vi "pp2_DAQwritePlayClick.vi"(0 "State In":T1={"Curr  tr"=0, "Curr (ms)"=0, "Cum (ms)"=0, "Run loop diff"=0, "Tone countdown (ms)"=0, "Countdown (ms)"=0, "Curr State"=enum."0 NULL", "Prev State"=enum."1 Habituation", "Null"=FALSE, "Sw"=FALSE, "Tone\nGate"=FALSE, "Stim"=FALSE, "Current DAQ DO Int"=0, "Current Loaded Trial"={"Trial Type Number"=1, "Trial Type"=enum."GO", "Trial Weight"=100, "Shock (mA)"=0.3, "Duration (ms)"=0.25, "Sound Type"=enum."04 FM Sweep", "Stim P1"=4000.0, "Stim P2"=0.0, "Stim P3"=0.0, "Stim P4"=2000.0}, "Next Trial (for display purposes)"={"Trial Type Number"=1, "Trial Type"=enum."GO", "Trial Weight"=100, "Shock (mA)"=0.3, "Duration (ms)"=0.25, "Sound Type"=enum."04 FM Sweep", "Stim P1"=4000.0, "Stim P2"=0.0, "Stim P3"=0.0, "Stim P4"=2000.0}, "Total trials memo"=0, "State start cum memo (ms)"=0, "Last dur jump time memo (ms)"=0, "Last dur shock time memo (ms)"=0, "Tone repeat memo (ms)"=0, "Webcam on"=FALSE, "Webcam recording"=FALSE} {"Current DAQ DO Int" format="%b"; "Next Trial (for display purposes)"."Shock (mA)" min=-1.0 max=5.0; "Next Trial (for display purposes)"."Trial Weight" step=1; "Next Trial (for display purposes)"."Duration (ms)" min=0.0 max=1.0; "Next Trial (for display purposes)"."Trial Type Number" min=1 step=1; "Current Loaded Trial"."Shock (mA)" min=-1.0 max=5.0; "Current Loaded Trial"."Trial Weight" step=1; "Current Loaded Trial"."Duration (ms)" min=0.0 max=1.0; "Current Loaded Trial"."Trial Type Number" min=1 step=1}, 1 "Daq config":T6={"Sound AO"="Dev2/ao0", "Shock intesity AO"="Dev1/ao1", "Code_LED DO"="Dev1/port1:2", "Switch DI"="Dev1/port0/line0:1", "Webcam"="cam0", "Sound AO task"="", "Sound card task"=0, "Shock intensity AO task"="", "Code_LED DO task"="", "Switch DI task"="", "AO <=> Sound card"=FALSE, "Sound card"=0, "sample rate"=8000.0, "Variable shock"=FALSE, "Webcam on"=FALSE, "Tone gate PFI"="/Dev1/PFI1", "Waveform memo"={"t0"=timestamp(0 s since 1904-01-01), "dt"=1.0, "Y"=[]}} {"sample rate" min=8000.0; "Sound card task" format="%.0x"}, 2 "Pre click \n(V)":dbl, 3 "error in (no error)":errorcluster) -> (8 "Daq config 2":T6={"Sound AO"="Dev2/ao0", "Shock intesity AO"="Dev1/ao1", "Code_LED DO"="Dev1/port1:2", "Switch DI"="Dev1/port0/line0:1", "Webcam"="cam0", "Sound AO task"="", "Sound card task"=0, "Shock intensity AO task"="", "Code_LED DO task"="", "Switch DI task"="", "AO <=> Sound card"=FALSE, "Sound card"=0, "sample rate"=8000.0, "Variable shock"=FALSE, "Webcam on"=FALSE, "Tone gate PFI"="/Dev1/PFI1", "Waveform memo"={"t0"=timestamp(0 s since 1904-01-01), "dt"=1.0, "Y"=[]}} {"sample rate" min=8000.0; "Sound card task" format="%.0x"}, 10 "error out":errorcluster)   [LabVIEW 2013]
uses:
  pp2_CTL_DaqConfig.ctl
  <vilib>/userdefined/High Color/IMAQdx.ctl
  <vilib>/sound2/lvsound2.llb/Sound Output Task ID.ctl
  pp2_CTL_StateInfo.ctl
  pp2_CTL_State.ctl
  pp2_Trial.ctl
  pp2_CTL_TrialType.ctl
  labolabo2/waveforms/WFTypes.ctl
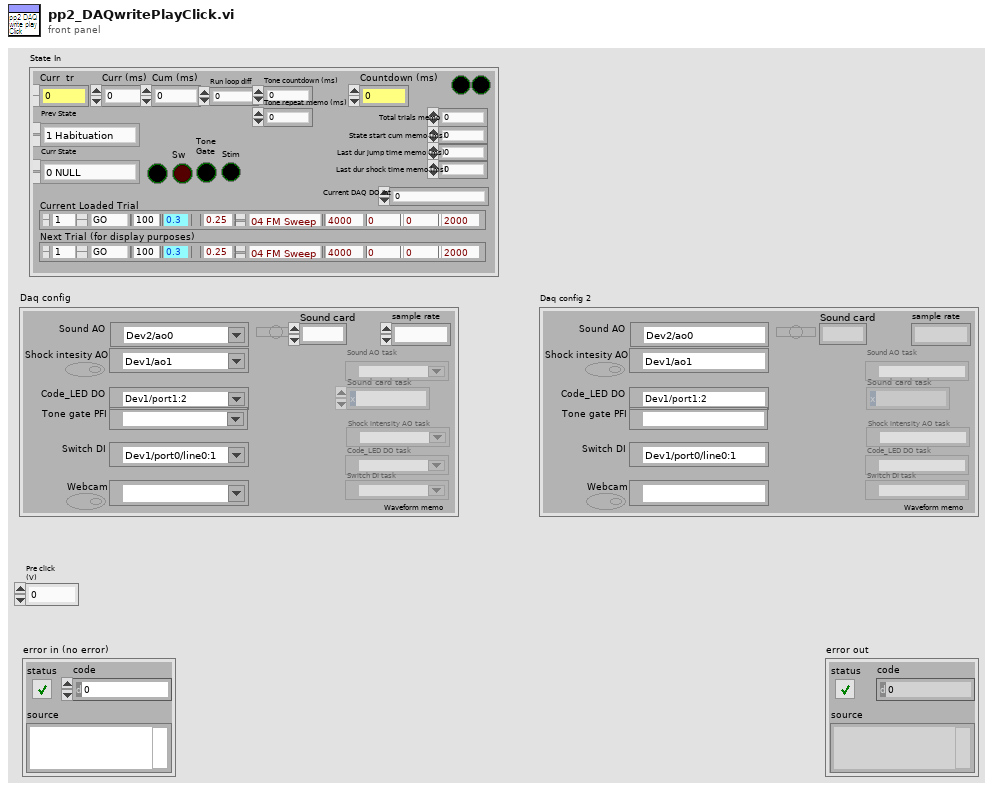
[diagram p1: front panel]
types:
  T1 = typedef "pp2_CTL_StateInfo.ctl" = cluster{"Curr  tr":u16, "Curr (ms)":u32, "Cum (ms)":i64, "Run loop diff":i64, "Tone countdown (ms)":i64, "Countdown (ms)":i64, "Curr State":T2, "Prev State":T2, "Null":bool, "Sw":bool, "Tone\nGate":bool, "Stim":bool, "Current DAQ DO Int":u16, "Current Loaded Trial":T3, "Next Trial (for display purposes)":T3, "Total trials memo":i64, "State start cum memo (ms)":i64, "Last dur jump time memo (ms)":i64, "Last dur shock time memo (ms)":i64, "Tone repeat memo (ms)":i64, "Webcam on":bool, "Webcam recording":bool}
  T2 = typedef "pp2_CTL_State.ctl" = enum8{"0 NULL", "1 Habituation", "2 (Load Trial)", "3 Stay Period", "4 Load Audio/Click Delay", "5 GO Trial", "6 GO Jumped", "7 GO Timeout", "8 NOGO Trial", "9 NOGO Jumped", "10 NOGO Timeout", "11 TEST Trial", "12 TEST Jumped", "13 TEST Timeout", "14 Intertrial Interval", "15 Done"}
  T3 = typedef "pp2_Trial.ctl" = cluster{"Trial Type Number":u8, "Trial Type":T4, "Trial Weight":u32, "Shock (mA)":dbl, "Duration (ms)":dbl, "Sound Type":T5, "Stim P1":dbl, "Stim P2":dbl, "Stim P3":dbl, "Stim P4":dbl}
  T4 = typedef "pp2_CTL_TrialType.ctl" = enum16{"OFF", "GO", "NOGO", "TEST"}
  T5 = typedef "WFTypes.ctl" = enum16{"00 NULL", "01 DC", "02 Noise", "03 Pure Tone", "04 FM Sweep"}
  T6 = typedef "pp2_CTL_DaqConfig.ctl" = cluster{"Sound AO":tag, "Shock intesity AO":tag, "Code_LED DO":tag, "Switch DI":tag, "Webcam":T7, "Sound AO task":refnum<k21>, "Sound card task":T8, "Shock intensity AO task":refnum<k21>, "Code_LED DO task":refnum<k21>, "Switch DI task":refnum<k21>, "AO <=> Sound card":bool, "Sound card":u32, "sample rate":dbl, "Variable shock":bool, "Webcam on":bool, "Tone gate PFI":tag, "Waveform memo":waveform(dbl)}
  T7 = typedef "IMAQdx.ctl" = refnum<k21>
  T8 = typedef "Sound Output Task ID.ctl" = u32
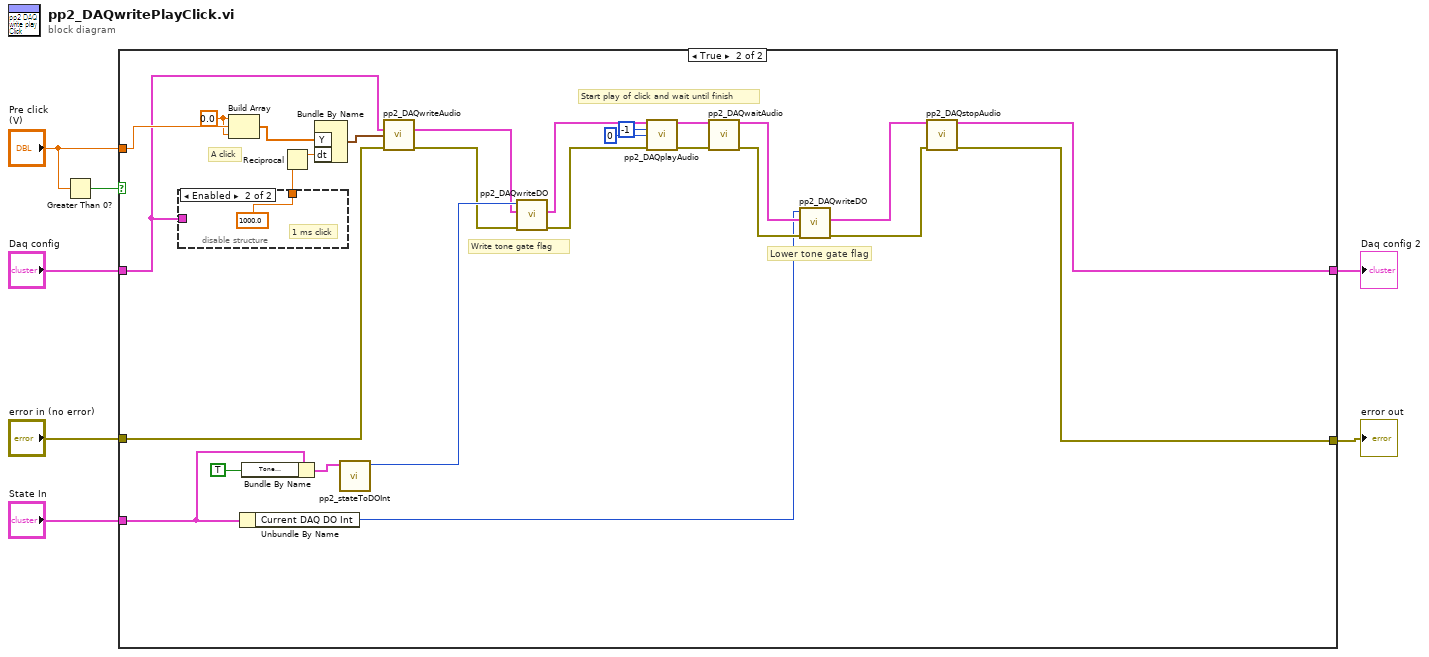
[diagram p0: block diagram]
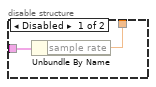
[diagram p3: hidden frame]
diagram:
  n1 = Greater Than 0?(x="Pre click \n(V)") -> (x > 0?=w3:bool)
  n2 = case shown="True" w3 {
    tunnel: "error in (no error)" -> [w8 w29]
    tunnel: [w8 w10] -> w6
    tunnel: [w9 w12] -> w5
    tunnel: "Daq config" -> [w9 w28]
    tunnel: "Pre click \n(V)" -> [_ w36]
    tunnel: "State In" -> [_ w34]
    frame False {
      # "If click amplitude is negative or zero, then just pass through without anything"
    }
    frame True {
      w35 = 0.0 ("element")
      # "Start play of click and wait until finish"
      # "Lower tone gate flag"
      # "Write tone gate flag"
      # "A click"
      n3 = disable-structure shown="Enabled" {
        disable-tunnel: [w38 1000.0 ("sample rate")] -> w31
        disable-tunnel: w28 -> [w37 _]
        frame Disabled {
          n4 = Unbundle By Name(w37) -> ("sample rate"=w38:dbl)
        }
        frame Enabled {
          # "1 ms click"
        }
      }
      n5 = Build Array(w35, w36, w35) -> (w33:dbl[])
      n6 = Unbundle By Name(w34) -> ("Current DAQ DO Int"=w16:u16)
      n7 = Bundle By Name(cluster=w34, "Tone\nGate"=TRUE ("Tone\nGate")) -> (w27:T1)
      n8 = Reciprocal(x=w31) -> (1/x=w32:dbl)
      n9 = Bundle By Name("Y"=w33, "dt"=w32) -> (w30:waveform(dbl))  [unwired: 1 in]
      n10 = call "pp2_stateToDOInt.vi"("State In"=w27) -> ("DAQ Output Int"=w25:u16)  [unwired: 10 in]
      n11 = call "pp2_DAQwriteAudio.vi"("Daq config In"=w28, "Waveform"=w30, "error in (no error)"=w29) -> ("Daq config Out"=w15:T6, "error out"=w14:errorcluster)  [unwired: 11 in]
      n12 = call "pp2_DAQwriteDO.vi"("error in (no error)"=w14, "Daq config"=w15, "DAQ Digital In"=w25) -> ("error out"=w23:errorcluster, "Daq config 2"=w24:T6)  [unwired: 7 in]
      n13 = call "pp2_DAQplayAudio.vi"("Daq config In"=w24, "Tone countdown (ms) In"=i64 -1, "Tone repeat memo"=i64 0, "error in (no error)"=w23) -> ("Daq config Out"=w20:T6, "error out"=w19:errorcluster)  [unwired: 9 in, 1 out]
      n14 = call "pp2_DAQwaitAudio.vi"("Daq config In"=w20, "error in (no error)"=w19) -> ("Daq config Out"=w17:T6, "error out"=w18:errorcluster)  [unwired: 12 in]
      n15 = call "pp2_DAQwriteDO.vi"("error in (no error)"=w18, "Daq config"=w17, "DAQ Digital In"=w16) -> ("error out"=w11:errorcluster, "Daq config 2"=w13:T6)  [unwired: 7 in]
      n16 = call "pp2_DAQstopAudio.vi"("Daq config In"=w13, "error in (no error)"=w11) -> ("Daq config Out"=w12:T6, "error out"=w10:errorcluster)  [unwired: 12 in]
    }
  }
  "error out" <- w6
  "Daq config 2" <- w5
